vi "Build Version.vi"(8 "Current Phase":T1, 9 "Revision":u32=1 min=1, 10 "Minor Revision":u16, 11 "Major Revision":u16) -> (3 "VI Version":string)   [LabVIEW 2014]
uses:
  TYPE_Version Status.ctl
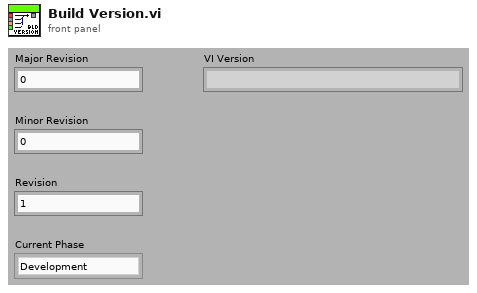
[diagram p1: front panel]
types:
  T1 = typedef "TYPE_Version Status.ctl" = enum16{"Development", "alpha", "beta", "Reviewed", "Bug", "Other"}
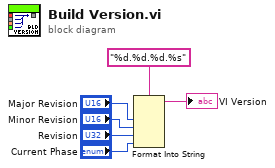
[diagram p0: block diagram]
diagram:
  n1 = Format Into String(format string="%d.%d.%d.%s" ("Author"), "Major Revision", "Minor Revision", "Revision", "Current Phase") -> (resulting string=→"VI Version":string)  [unwired: 2 in, 1 out]
